vi "RTS Relay 1 Startup.vi"(11 "Station 1-8 Data in":T1 {"Station Slide"."Chamber 1-1"."Start Time" format="%<%X\n%x>T"; "Station Slide"."Chamber 1-1"."End Time" format="%<%X\n%x>T"; "Station Slide"."Time Count (s)" format="%.2f"; "Station Cab"."Chamber 1-1"."Start Time" format="%<%X\n%x>T"; "Station Cab"."Chamber 1-1"."End Time" format="%<%X\n%x>T"; "Station Cab"."Time Count (s)" format="%.2f"; "Station Freezer"."Chamber 1-1"."Start Time" format="%<%X\n%x>T"; "Station Freezer"."Chamber 1-1"."End Time" format="%<%X\n%x>T"; "Station Freezer"."Time Count (s)" format="%.2f"}) -> (3 "Run Door Ops":bool)   [LabVIEW 2016]
uses:
  Type Definitions/RTS Station Relay Ops.ctl
  Type Definitions/RTS Door Opener Indicator.ctl
  Type Definitions/RTS Door Ops Client.ctl
  Type Definitions/RTS Door Opening Schedule.ctl
  Type Definitions/RTS Door Ops Sequence.ctl
panel:
  # "Chamber Conditions:"
  # "Chamber Conditions:"
  # "Chamber Conditions:"
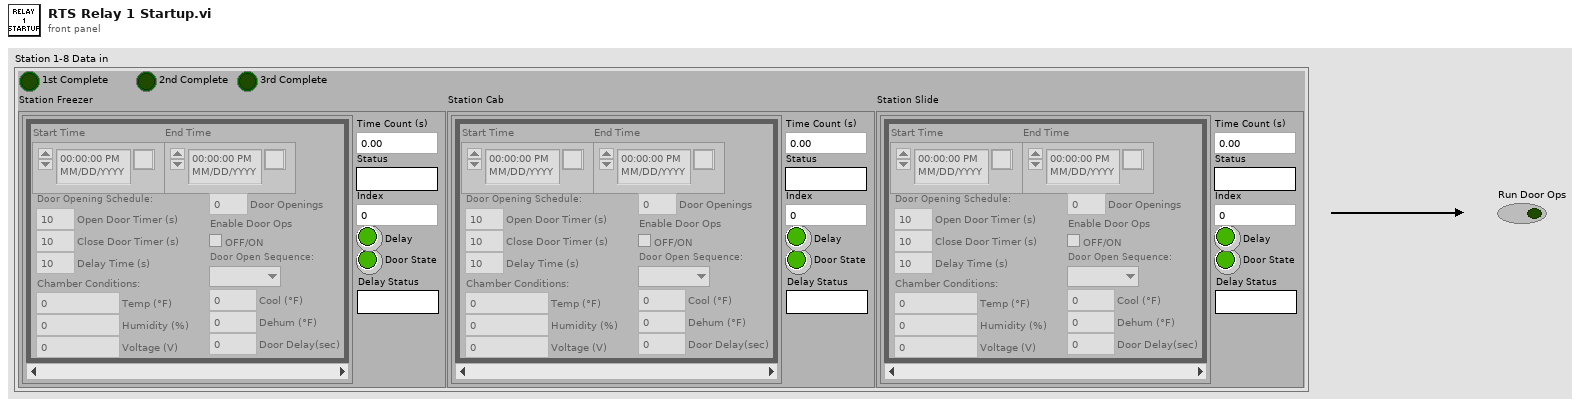
[diagram p1: front panel]
types:
  T1 = typedef "RTS Station Relay Ops.ctl" = cluster{"Station Freezer":T2, "Station Cab":T2, "Station Slide":T2, "1st Complete":bool, "2nd Complete":bool, "3rd Complete":bool}
  T2 = typedef "RTS Door Opener Indicator.ctl" = cluster{"Time Count (s)":dbl, "Status":string, "Door State":bool, "Delay":bool, "Chamber 1-1":T3[], "Index":i32, "Delay Status":string}
  T3 = typedef "RTS Door Ops Client.ctl" = cluster{"End Time":timestamp, "Start Time":timestamp, "Door Opening Schedule:":T4, "Enable Door Ops":bool, "Door Openings":u32, "Temp (°F)":dbl, "Humidity (%)":dbl, "Voltage (V)":dbl, "Door Open Sequence:":T5, "Door Delay(sec)":dbl, "Dehum (°F)":dbl, "Cool (°F)":dbl}
  T4 = typedef "RTS Door Opening Schedule.ctl" = cluster{"Open Door Timer (s)":dbl, "Delay Time (s)":dbl, "Close Door Timer (s)":dbl}
  T5 = typedef "RTS Door Ops Sequence.ctl" = enum16{"", "1st", "2nd", "3rd"}
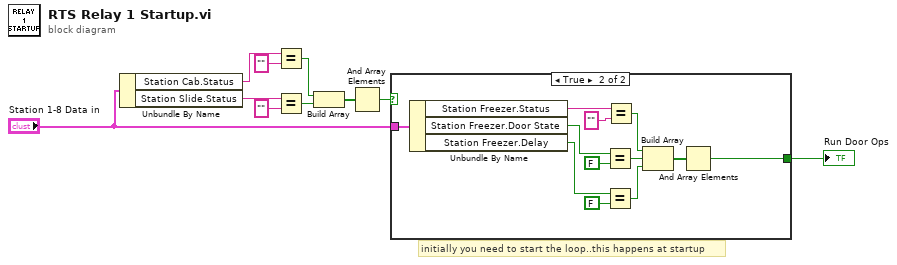
[diagram p0: block diagram]
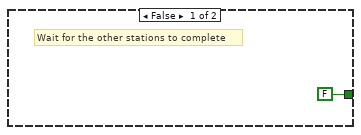
[diagram p2: hidden frame]
diagram:
  # "initially you need to start the loop..this happens at startup"
  n1 = Unbundle By Name("Station 1-8 Data in") -> ("Station Cab.Status"=w6:string, "Station Slide.Status"=w5:string)
  n2 = Equal?(x=w6, y="") -> (x = y?=w7:bool)
  n3 = Equal?(x=w5, y="") -> (x = y?=w8:bool)
  n4 = Build Array(w7, w8) -> (w9:bool[])
  n5 = And Array Elements(Boolean array=w9) -> (logical AND=w10:bool)
  n6 = case shown="False" w10 {
    tunnel: [FALSE w13] -> w1
    tunnel: "Station 1-8 Data in" -> [_ w12]
    frame False {
      # "Wait for the other stations to complete"
    }
    frame True {
      n7 = Unbundle By Name(w12) -> ("Station Freezer.Status"=w16:string, "Station Freezer.Door State"=w15:bool, "Station Freezer.Delay"=w14:bool)
      n8 = Equal?(x=w15, y=FALSE) -> (x = y?=w19:bool)
      n9 = Equal?(x=w14, y=FALSE) -> (x = y?=w18:bool)
      n10 = Equal?(x=w16, y="") -> (x = y?=w20:bool)
      n11 = Build Array(w20, w19, w18) -> (w17:bool[])
      n12 = And Array Elements(Boolean array=w17) -> (logical AND=w13:bool)
    }
  }
  "Run Door Ops" <- w1
